vi "Memory.Pointer.Read All (unsafe).vi"(8 "error in (no error)":errorcluster, 10 "buffer in":string, 11 "Pointer in":refnum<class "Memory.Pointer.lvclass">) -> (0 "error out":errorcluster, 2 "buffer out":string, 3 "Pointer out":refnum<class "Memory.Pointer.lvclass">)   [LabVIEW 2016, in "LabVIEW Memory Manager.lvlib" / "Memory.Pointer.lvclass"]
uses:
  Memory.Pointer.lvclass
  Memory.Pointer.lvclass/Memory.Pointer.ctl
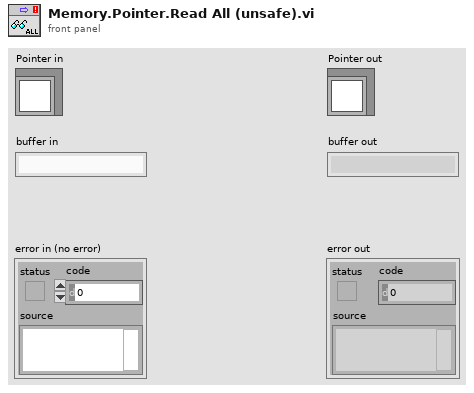
[diagram p1: front panel]
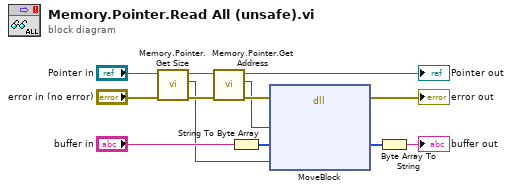
[diagram p0: block diagram]
diagram:
  n1 = call "Memory.Pointer.Get Size.vi"("error in (no error)"="error in (no error)", "Pointer in"="Pointer in") -> ("error out"=w8:errorcluster, "size"=w4:i64, "Pointer out"=w7:refnum<class "Memory.Pointer.lvclass">)  [unwired: 7 in]
  n2 = call "Memory.Pointer.Get Address.vi"("error in (no error)"=w8, "Pointer in"=w7) -> ("error out"=w6:errorcluster, "address"=w3:u64, "Pointer out"=→"Pointer out":refnum<class "Memory.Pointer.lvclass">)  [unwired: 7 in]
  n3 = String To Byte Array(string="buffer in") -> (unsigned byte array=w2:u8[])
  n4 = dll-call lib="LabVIEW" fn="MoveBlock"(error in=w6, "src pointer"=w3, "dst pointer"=w2, "size"=w4) -> (error out=→"error out":errorcluster, "dst pointer"=w12:u8[])  [unwired: 5 in, 1 out]
  n5 = Byte Array To String(unsigned byte array=w12) -> (string=→"buffer out":string)
